vi "StartDataCollectionObsolete.vi"(8 "error in (no error)":errorcluster, 9 "Period (msec)":dbl=1.0, 10 "Points":i32=1000, 11 "controller in":refnum<k24>) -> (0 "error out":errorcluster, 3 "controller out":refnum<k24>)   [LabVIEW 2010]
uses:
  c:/aerotech/controller/dev/A3200/pc/labview/2010/bin/Aerotech.A3200.dll
  bin/Aerotech.A3200.dll
  c:/aerotech/controller/dev/A3200/pc/labview/2010/bin/Aerotech.A3200.LabVIEW.dll
  bin/Aerotech.A3200.LabVIEW.dll
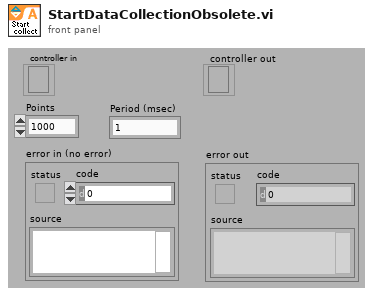
[diagram p1: front panel]
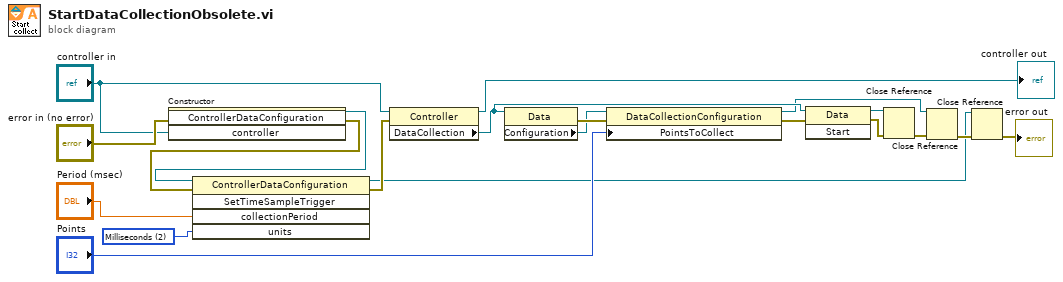
[diagram p0: block diagram]
diagram:
  w9 = 2 items=["Seconds", "Minutes", "Milliseconds", "Microseconds"] ("units")
  n1 = constructor class="ControllerDataConfiguration"(error in="error in (no error)", "controller"="controller in") -> (reference out=w11:refnum<k24>, error out=w12:errorcluster)  [unwired: 2 in, 2 out]
  n2 = invoke class="ControllerDataConfiguration" method="SetTimeSampleTrigger"(reference=w11, error in=w12, "collectionPeriod"="Period (msec)", "units"=w9) -> (reference out=w2:refnum<k24>, error out=w8:errorcluster)  [unwired: 1 in, 3 out]
  n3 = property class="Controller"(reference="controller in", error in=w8) -> (reference out=→"controller out":refnum<k24>, "DataCollection"=w20:refnum<k24>)  [unwired: 1 out]
  n4 = property class="Data"(reference=w20) -> (error out=w16:errorcluster, "Configuration"=w15:refnum<k24>)  [unwired: 1 in, 1 out]
  n5 = property class="DataCollectionConfiguration"(reference=w15, error in=w16, "PointsToCollect"="Points") -> (reference out=w4:refnum<k24>, error out=w17:errorcluster)
  n6 = invoke class="Data" method="Start"(reference=w20, error in=w17) -> (reference out=w5:refnum<k24>, error out=w6:errorcluster)  [unwired: 1 in, 1 out]
  n7 = Close Reference(reference=w5, error in (no error)=w6) -> (error out=w18:errorcluster)
  n8 = Close Reference(reference=w4, error in (no error)=w18) -> (error out=w3:errorcluster)
  n9 = Close Reference(reference=w2, error in (no error)=w3) -> (error out=→"error out":errorcluster)
